vi "MPM_Logging_Stop.vi"(8 "error in (no error)":errorcluster, 11 ".NET Reference in":refnum<k24>) -> (0 "error out":errorcluster, 3 "Reference out":refnum<k24>)   [LabVIEW 2017]
uses:
  C:/Users/Ssantec_Test/Documents/Instrument_DLL_Sample_Labview_20220902_Ver1.2.2/DLL/x86/InstrumentDLL.dll
  DLL/x86/InstrumentDLL.dll
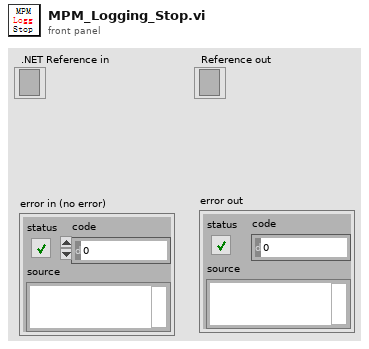
[diagram p1: front panel]
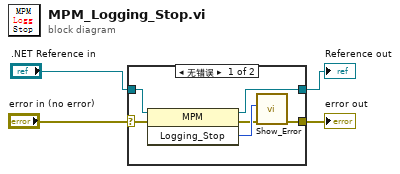
[diagram p0: block diagram]
diagram:
  n1 = case shown="无错误" "error in (no error)" {
    selector: "error in (no error)" -> [w10 w12]
    tunnel: ".NET Reference in" -> [w8 w11]
    tunnel: [w5 w12] -> w2
    tunnel: [w9 w11] -> w1
    frame No Error {
      n2 = invoke class="MPM" method="Logging_Stop"(reference=w8, error in=w10) -> (reference out=w9:refnum<k24>, error out=w6:errorcluster, "Logging_Stop"=w7:i32)  [unwired: 1 in]
      n3 = call "Show_Error.vi"("error in (no error)"=w6, "Error"=w7) -> ("error out"=w5:errorcluster)  [unwired: 9 in]
    }
    frame Error {
    }
  }
  "Reference out" <- w1
  "error out" <- w2
